vi "MixedGraphView(old).vi"() -> ()   [LabVIEW 2014]
uses:
  GlobalData/GlobalData.vi
panel:
  out "ミックスドシグナルグラフ":waveform(dbl)[](graph)
  # "右クリック→カーソルを作成→複数プロット。さらに右クリック→監視→全てのプロット"
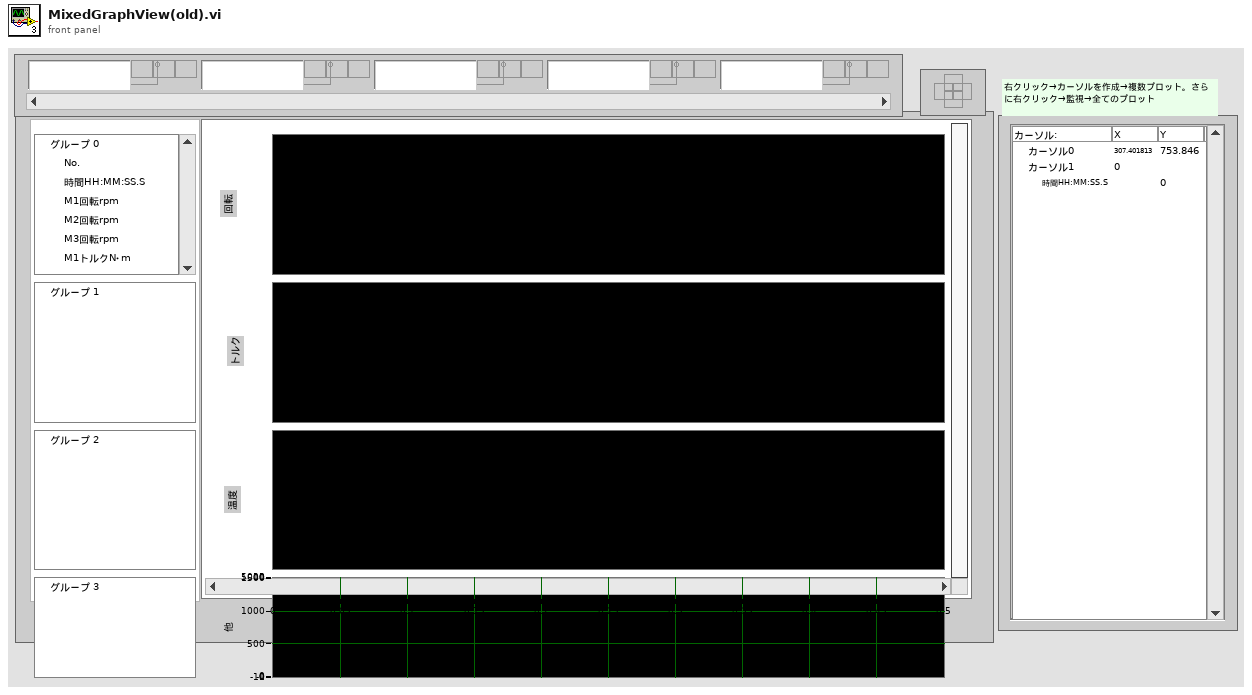
[diagram p1: front panel]
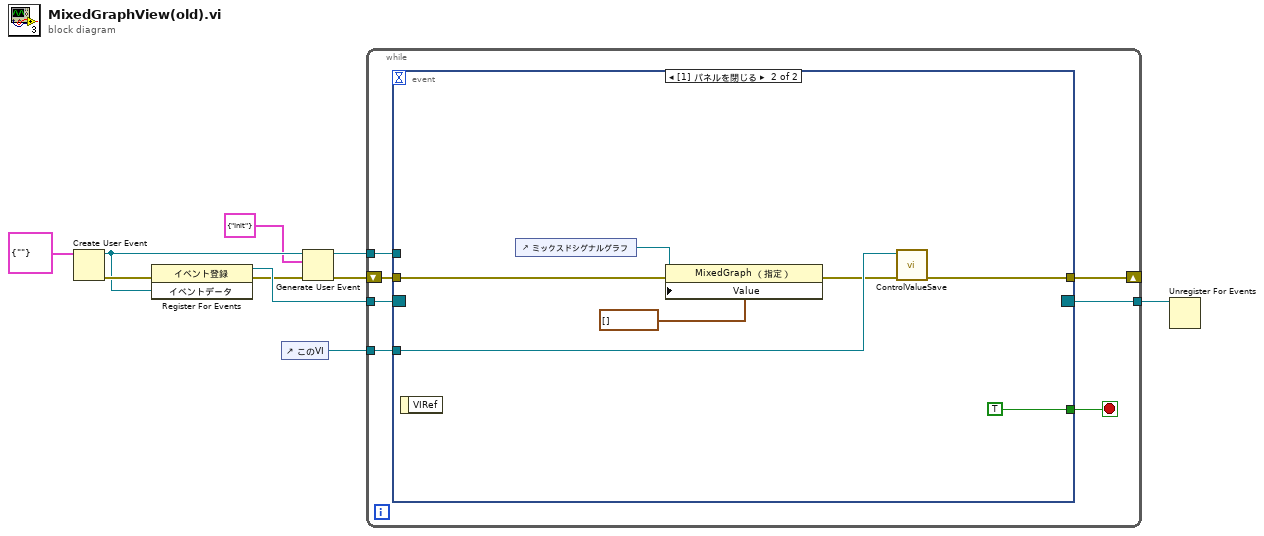
[diagram p0: block diagram]
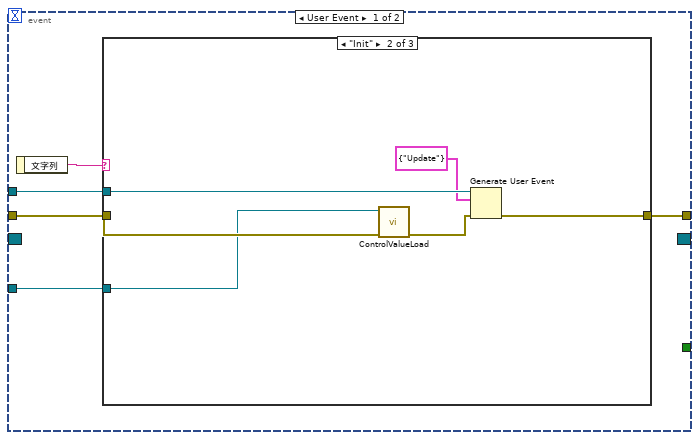
[diagram p2: hidden frame]
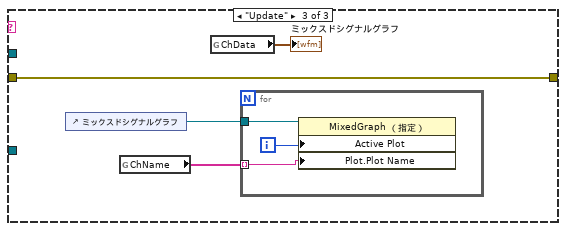
[diagram p4: hidden frame]
diagram:
  n1 = Create User Event(user event datatype=cluster{"文字列":string} {"文字列"=""} ("イベントデータ")) -> (user event=w7:refnum<user-event>, error out=w8:errorcluster)  [unwired: 1 in]
  n2 = register-events(error in=w8, w7) -> (reference out=w10:refnum<event-registration>, error out=w6:errorcluster)  [unwired: 1 in]
  n3 = control-ref of="このVI"() -> (w1:refnum<vi>)
  n4 = Generate User Event(user event=w7, event data cluster=cluster{"文字列":string} {"文字列"="Init"} ("イベントデータ"), error in=w6) -> (user event out=w2:refnum<user-event>, error out=w5:errorcluster)  [unwired: 1 in]
  n5 = while {
    tunnel: w10 -> [w16]
    tunnel: [w15] -> w3
    tunnel: w2 -> [w14]
    tunnel: w1 -> [w13]
    shift-right: [w11] -> _
    shift-left: w5 -> [w12]
    stop <- w17 stop-if-true
    n6 = event shown="[1] パネルを閉じる" {
      selector: w16 -> [_ _]
      dyn-events: [_ _] -> w15
      timeout: _ -> [_ _]
      tunnel: [_ TRUE] -> w17
      tunnel: w14 -> [w21 _]
      tunnel: w13 -> [w20 w42]
      tunnel: w12 -> [w19 w38]
      tunnel: [w18 w37] -> w11
      event User Event {
        n7 = event-data() -> ("文字列"=w22:string)  [unwired: 1 in]
        n8 = case shown="\"Init\"" w22 {
          tunnel: w21 -> [_ w29 _]
          tunnel: w20 -> [_ w24 _]
          tunnel: w19 -> [w23 w26 w32]
          tunnel: [w23 w25 w32] -> w18
          frame Default {
          }
          frame "Init" {
            n9 = call "ControlValueLoad.vi"("err(in)"=w26, "VI refnum"=w24) -> ("err(out)"=w27:errorcluster)  [unwired: 9 in]
            n10 = Generate User Event(user event=w29, event data cluster=cluster{"文字列":string} {"文字列"="Update"} ("イベントデータ"), error in=w27) -> (error out=w25:errorcluster)  [unwired: 1 in, 1 out]
          }
          frame "Update" {
            n11 = control-ref of="ミックスドシグナルグラフ"() -> (w31:refnum<vi>)
            n12 = global read "GlobalData.vi" "ChName"() -> (w30:string[])
            n13 = global read "GlobalData.vi" "ChData"() -> (→"ミックスドシグナルグラフ":waveform(dbl)[])
            n14 = for {
              tunnel: w31 -> [w36]
              tunnel: w30 -> [w34] mode=indexing
              i -> [w35]
              n15 = property class="MixedGraph （指定）"(reference=w36, "Active Plot"=w35, "Plot.Plot Name"=w34) -> ()  [unwired: 1 in, 2 out]
            }
          }
        }
      }
      event Panel Close {
        n16 = event-data() -> ()  [unwired: 1 in, 1 out]
        n17 = control-ref of="ミックスドシグナルグラフ"() -> (w41:refnum<vi>)
        n18 = property class="MixedGraph （指定）"(reference=w41, error in=w38, "Value"=waveform(dbl)[] [] ("値")) -> (error out=w39:errorcluster)  [unwired: 1 out]
        n19 = call "ControlValueSave.vi"("err(in)"=w39, "VI refnum"=w42) -> ("err(out)"=w37:errorcluster)  [unwired: 9 in]
      }
    }
  }
  n20 = Unregister For Events(event registration refnum=w3) -> ()  [unwired: 1 in, 1 out]
